vi "niDTS BT INSTR TX Close.vi"(8 "error in (no error)":errorcluster, 11 "niDTS BT INSTR TX in":refnum<class "niDTS BT INSTR TX.lvclass">) -> (0 "error out":errorcluster, 3 "niDTS BT INSTR TX out":refnum<class "niDTS BT INSTR TX.lvclass">)   [LabVIEW 2015, in "niDTS BT.lvlib" / "niDTS BT INSTR TX.lvclass"]
uses:
  niDTS BT INSTR TX.lvclass
  niDTS BT INSTR TX.lvclass/niDTS BT INSTR TX.ctl
  RiviInstDriver/InstDriver/Objects/InstDriver.lvclass
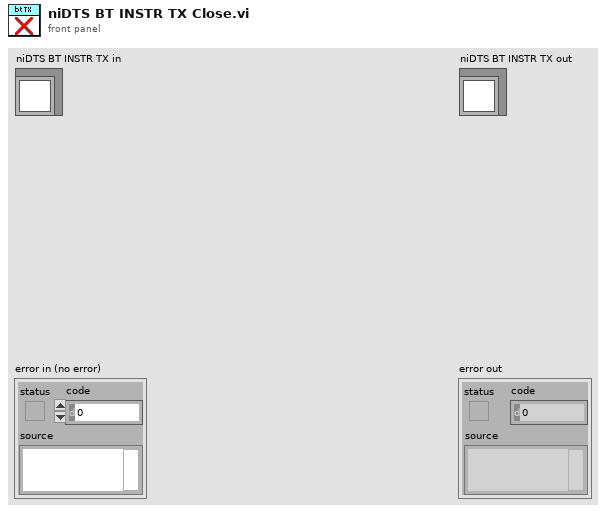
[diagram p1: front panel]
types:
  T1 = typedef "niRfsaBT.lvclass/niRfsaBT INC Handle.ctl" = refnum<data-value>
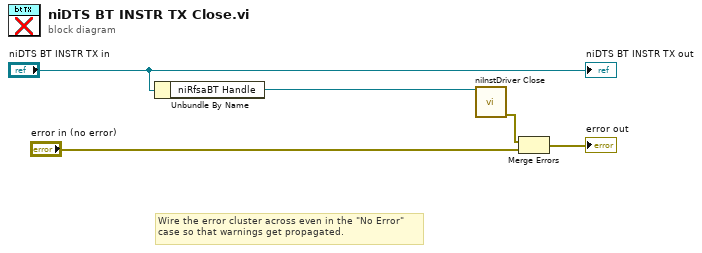
[diagram p0: block diagram]
diagram:
  # "Wire the error cluster across even in the \"No Error\"\ncase so that warnings get propagated."
  n1 = Unbundle By Name("niDTS BT INSTR TX in") -> ("niRfsaBT Handle"=w3:T1)
  n2 = call "niInstDriver Close.vi"("InstDriver Handle in"=w3) -> ("error out"=w2:errorcluster)  [unwired: 14 in]
  n3 = Merge Errors(w2, "error in (no error)") -> (→"error out":errorcluster)
  "niDTS BT INSTR TX out" <- "niDTS BT INSTR TX in"
